vi "Configure SMU Output Resistance.vi"(7 "Resistance Level (0.0 ohms)":dbl format="%^.3e", 8 "error in (no error)":errorcluster {"code" format="%.0x"}, 9 "Enable Output Resistance (False)":bool, 10 "Channel Name (1)":string="1", 11 "VISA resource name":refnum<visa-resource-name>) -> (0 "error out":errorcluster {"code" format="%.0x"}, 3 "VISA resource name out":refnum<visa-resource-name>)   [LabVIEW 2016, in "Agilent N6700 Series.lvlib"]
doc: "Sets the state of the output resistance and resistance level on the specified channels.\n\n<b>Notes:</b>\n(1) This VI only applies to the N6781A, N6785A and N679xA model.\n(2) The output protection priority must be set to voltage in <b>Configure Output Regulation.vi</b>."
uses:
  <instrlib>/Agilent N6700 Series/Agilent N6700 Series.lvlib
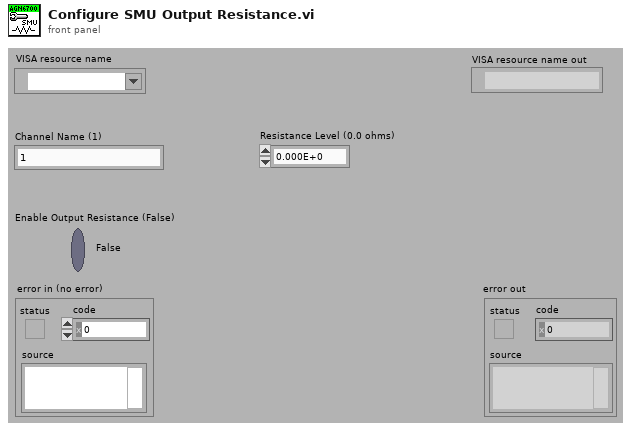
[diagram p1: front panel]
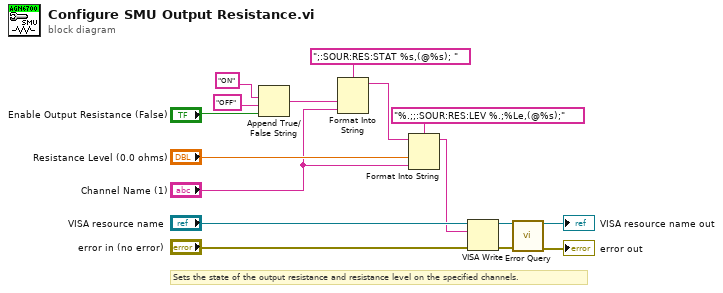
[diagram p0: block diagram]
diagram:
  # "Sets the state of the output resistance and resistance level on the specified channels."
  n1 = Append True/False String(1:"Enable Output Resistance (False)", 2:"OFF", 3:"ON") -> (0:w7:string)  [unwired: 1 in]
  n2 = Format Into String(format string=";:SOUR:RES:STAT %s,(@%s); ", w7, "Channel Name (1)") -> (resulting string=w10:string)  [unwired: 2 in, 1 out]
  n3 = Format Into String(format string="%.;;:SOUR:RES:LEV %.;%Le,(@%s);", initial string=w10, "Resistance Level (0.0 ohms)", "Channel Name (1)") -> (resulting string=w2:string)  [unwired: 1 in, 1 out]
  n4 = VISA Write(VISA resource name="VISA resource name", write buffer=w2, error in (no error)="error in (no error)") -> (VISA resource name out=w12:refnum<visa-resource-name>, error out=w11:errorcluster)  [unwired: 1 out]
  n5 = call <instrlib>:"Error Query.vi"("VISA resource name"=w12, "error in (no error)"=w11) -> ("VISA resource name out"=→"VISA resource name out":refnum<visa-resource-name>, "error out"=→"error out":errorcluster)  [unwired: 10 in, 2 out]
